vi "FindString.vi"(9 "offset past match in":i32, 10 "FnR":T1, 11 "String":string) -> (2 "offset past match out":i32, 3 "Array":T2[](array[typedef]), 4 "# hits":i32)   [LabVIEW 2022 SP3]
uses:
  <vilib>/Utility/miscctls.llb/LVSelectionTypeDef.ctl
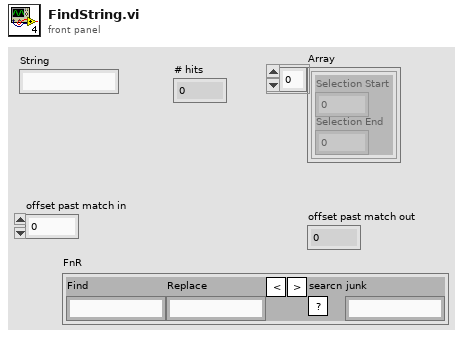
[diagram p1: front panel]
types:
  T1 = cluster{"Find":string, "Replace":string, "back":bool, "forward":bool, "searcn":bool, "junk":string}
  T2 = typedef "LVSelectionTypeDef.ctl" = cluster{"Selection Start":u32, "Selection End":u32}
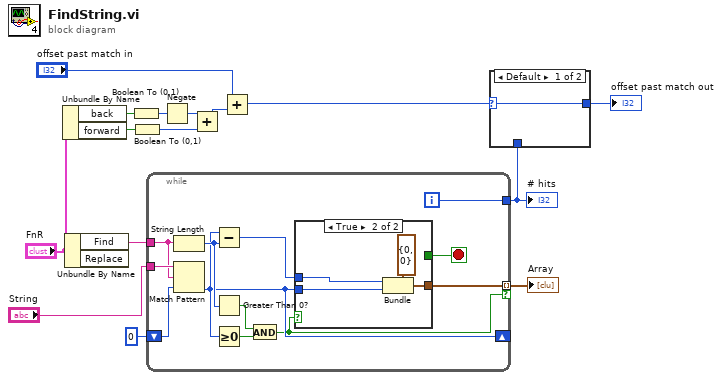
[diagram p0: block diagram]
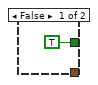
[diagram p3: hidden frame]
diagram:
  n1 = Unbundle By Name("FnR") -> ("back"=w10:bool, "forward"=w9:bool)
  n2 = Unbundle By Name("FnR") -> ("Find"=w13:string)  [unwired: 1 out]
  n3 = Boolean To (0,1)(Boolean=w10) -> (0, 1=w8:i16)
  n4 = Boolean To (0,1)(Boolean=w9) -> (0, 1=w6:i16)
  n5 = while {
    tunnel: "String" -> [w26]
    tunnel: w13 -> [w23]
    shift-right: [w21] -> _
    shift-left: 0 ("offset past match") -> [w20]
    tunnel: [w18] -> w15 mode=indexing if=w17
    tunnel: [w16] -> w1
    i -> [w16]
    stop <- w19 stop-if-true
    n6 = String Length(string=w23) -> (length=w22:i32)
    n7 = Match Pattern(string=w26, regular expression=w23, offset (0)=w20) -> (offset past match=w21:i32)  [unwired: 3 out]
    n8 = Subtract(x=w21, y=w22) -> (x-y=w27:i32)
    n9 = Greater Than 0?(x=w22) -> (x > 0?=w25:bool)
    n10 = Greater Or Equal To 0?(x=w21) -> (x >= 0?=w24:bool)
    n11 = And(x=w25, y=w24) -> (x .and. y?=w17:bool)
    n12 = case shown="True" w17 {
      tunnel: w27 -> [_ w32]
      tunnel: w21 -> [_ w30]
      tunnel: [TRUE _] -> w19
      tunnel: [_ w29] -> w18
      frame False {
      }
      frame True {
        n13 = Bundle(cluster=T2 {"Selection Start"=0, "Selection End"=0} ("Text.Selection"), "Selection Start"=w32, "Selection End"=w30) -> (w29:T2)
      }
    }
  }
  "Array" <- w15
  "# hits" <- w1
  n14 = Negate(x=w8) -> (-x=w7:i16)
  n15 = Add(x=w7, y=w6) -> (x+y=w5:i16)
  n16 = Add(x="offset past match in", y=w5) -> (x+y=w3:i32)
  n17 = case shown="Default" w3 {
    selector: w3 -> [w33 _]
    tunnel: [w33 w34] -> w2
    tunnel: w1 -> [_ w34]
    frame Default {
    }
    frame 0 {
    }
  }
  "offset past match out" <- w2
